vi "Record Best Solution.vi"(8 "error in (no error)":errorcluster, 9 "Generation Number":i32, 10 "GA.lvclass":refnum<class "GA.lvclass">, 11 "OSSP_Problem in":refnum<class "OSSP_Problem.lvclass">) -> (0 "error out":errorcluster, 1 "Best Fitness In Population":u16, 2 "GA out":refnum<class "GA.lvclass">, 3 "OSSP_Problem out":refnum<class "OSSP_Problem.lvclass">)   [LabVIEW 2013]
uses:
  Classes/GA.lvclass
  Classes/OSSP_Problem.lvclass
  Classes/OSSP_Problem.lvclass/OSSP_Problem.ctl
  Classes/GA.lvclass/GA.ctl
  Classes/GA_Class/Controls/Solution_GA.ctl
  Classes/GA_Class/Find Best Solution In Population.vi
  Classes/Scheduler_Class/Operation to Machine Job Tuple.vi
  <vilib>/Analysis/baseanly.llb/Mean.vi
  <vilib>/Analysis/baseanly.llb/Mean (DBL).vi
  Classes/Scheduler.lvclass
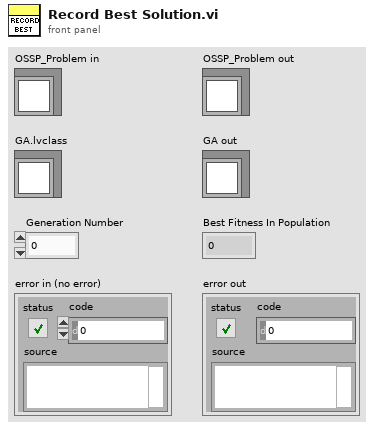
[diagram p1: front panel]
types:
  T1 = typedef "Solution_GA.ctl" = cluster{"Schedule":u16[], "Fitness":u16, "Fitness Valid?":bool}
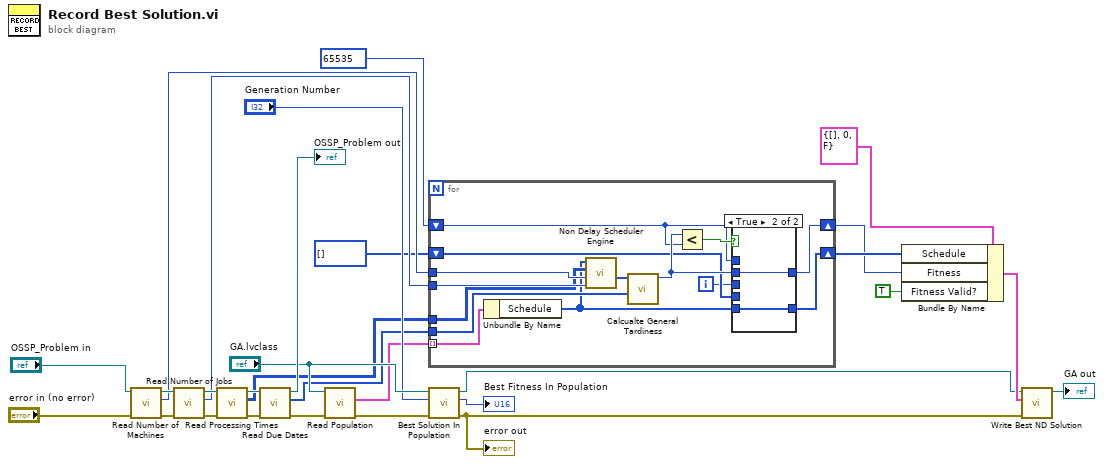
[diagram p0: block diagram]
diagram:
  n1 = call "Read Number of Machines.vi"("error in (no error)"="error in (no error)", "OSSP_Problem in"="OSSP_Problem in") -> ("error out"=w17:errorcluster, "Number of Machines"=w13:i32, "OSSP_Problem out"=w20:refnum<class "OSSP_Problem.lvclass">)  [unwired: 7 in]
  n2 = call "Read Number of Jobs.vi"("error in (no error)"=w17, "OSSP_Problem in"=w20) -> ("error out"=w16:errorcluster, "Number of Jobs"=w12:i32, "OSSP_Problem out"=w19:refnum<class "OSSP_Problem.lvclass">)  [unwired: 7 in]
  n3 = call "Read Processing Times.vi"("error in (no error)"=w16, "OSSP_Problem in"=w19) -> ("error out"=w15:errorcluster, "Processing Times"=w11:u16[][], "OSSP_Problem out"=w18:refnum<class "OSSP_Problem.lvclass">)  [unwired: 7 in]
  n4 = call "Read Due Dates.vi"("error in (no error)"=w15, "OSSP_Problem in"=w18) -> ("error out"=w14:errorcluster, "Due Dates"=w10:u16[], "OSSP_Problem out"=→"OSSP_Problem out":refnum<class "OSSP_Problem.lvclass">)  [unwired: 7 in]
  n5 = call "Read Population.vi"("error in (no error)"=w14, "GA in"="GA.lvclass") -> ("error out"=w9:errorcluster, "Population"=w21:T1[])  [unwired: 7 in, 1 out]
  n6 = for {
    tunnel: w21 -> [w43] mode=indexing
    tunnel: w13 -> [w41]
    tunnel: w12 -> [w40]
    tunnel: w11 -> [w39]
    tunnel: w10 -> [w38]
    shift-right: [w35] -> w4
    shift-left: u16 65535 -> [w34]
    shift-right: [w32] -> w5
    shift-left: u16[] [] ("Schedule") -> [w33]
    i -> [w31]
    n7 = Unbundle By Name(w43) -> ("Schedule"=w30:u16[])
    n8 = call "Non Delay Scheduler Engine.vi"("Number of  Jobs"=w40, "Number of Machines"=w41, "Processing Times"=w39, "Schedule"=w30) -> ("Job Completion Times"=w42:u16[])  [unwired: 2 in, 5 out]
    n9 = call "Calcualte General Tardiness.vi"("Due Dates"=w38, "Job Completion Times"=w42) -> ("Total Tardiness (U16)"=w36:u16)  [unwired: 9 in]
    n10 = Less?(x=w36, y=w34) -> (x < y?=w37:bool)
    n11 = case shown="True" w37 {
      tunnel: w36 -> [_ w47]
      tunnel: [w45 w47] -> w35
      tunnel: w34 -> [w45 _]
      tunnel: w33 -> [w44 _]
      tunnel: [w44 w46] -> w32
      tunnel: w31 -> [_ _]
      tunnel: w30 -> [_ w46]
      frame False {
      }
      frame True {
      }
    }
  }
  n12 = call "Best Solution In Population.vi"("error in (no error)"=w9, "Generation Number"="Generation Number", "GA in"="GA.lvclass") -> ("error out"=w28:errorcluster, "Best Fitness"=→"Best Fitness In Population":u16, "GA out"=w1:refnum<class "GA.lvclass">)  [unwired: 6 in]
  "error out" <- w28
  n13 = Bundle By Name(cluster=T1 {"Schedule"=[], "Fitness"=0, "Fitness Valid?"=FALSE} ("Solution"), "Schedule"=w5, "Fitness"=w4, "Fitness Valid?"=TRUE) -> (w3:T1)
  n14 = call "Write Best ND Solution.vi"("error in (no error)"=w28, "Solution"=w3, "GA in"=w1) -> ("GA out"=→"GA out":refnum<class "GA.lvclass">)  [unwired: 7 in, 1 out]
